vi "CR-导丝纤维毛发检测3参数读取.vi"(7 "error in (no error)":errorcluster caption="错误输入（无错误）", 10 "基路径":path) -> (0 "error out":errorcluster caption="错误输出", 1 "导丝纤维毛发检测3参数":T2={"Max Number"=11.0, "Curve Extraction Settings "={"Extraction Mode"=0, "Edge Threshold"=25, "Edge Filter Size"=1, "Min Length"=19, "Row Search Step Size"=5, "Col Search Step Size"=5, "Max Endpoint Gap"=10, "Closed"=FALSE, "Subpixel"=FALSE}, "Color Mode (Histogram 1)"=0, "Range (Threshold 1)"={"Lower value"=62.0, "Upper value"=255.0}, "Clamp Settings (Max Clamp 1)"={"Angle Range (+/-)"=10.0, "Edge Polarity"={"Start"=0, "End"=0}}, "Settings (Clamp (Rake) 1)"={"Contrast"=6, "Filter width"=5, "Steepness"=2, "Subsampling Ratio"=5, "Show Search Area"=TRUE, "Show Search Lines"=TRUE, "Show Edges Found"=TRUE, "Show Result"=TRUE}} {"Clamp Settings (Max Clamp 1)"."Edge Polarity"."Start" items=["Any", "Rising", "Falling"]; "Clamp Settings (Max Clamp 1)"."Edge Polarity"."End" items=["Any", "Rising", "Falling"]; "Color Mode (Histogram 1)" items=["RGB", "HSL", "HSV", "HSI"]; "Curve Extraction Settings"."Extraction Mode" items=["Normal", "Uniform Regions"]; "Curve Extraction Settings"."Edge Filter Size" items=["Fine", "Normal", "Contour Tracing"]; "Curve Extraction Settings"."Max Endpoint Gap" min=0; "Curve Extraction Settings"."Col Search Step Size" min=1 max=255 step=1; "Curve Extraction Settings"."Row Search Step Size" min=1 max=255 step=1; "Curve Extraction Settings"."Min Length" min=0; "Curve Extraction Settings"."Edge Threshold" min=1 max=350 step=1}, 2 "导丝纤维毛发检测3基础参数":T3={"IsNorImage"=TRUE, "Exposure Values"=100289, "ImagePath"=path "C:/Users/hedongpo/Desktop/514-hdp/Alignment Assemble System/Test Picture/B/3.bmp"} caption="参数界面" {"Exposure Values" scale=0.0..200000.0})   [LabVIEW 2017]
uses:
  <vilib>/vision/Pattern Matching.llb/IMAQ Curve Parameters.ctl
  <vilib>/Utility/xml.llb/Read From XML File(string).vi
  Global System.vi
panel:
  # "UI电源线反面标签1基础参数"
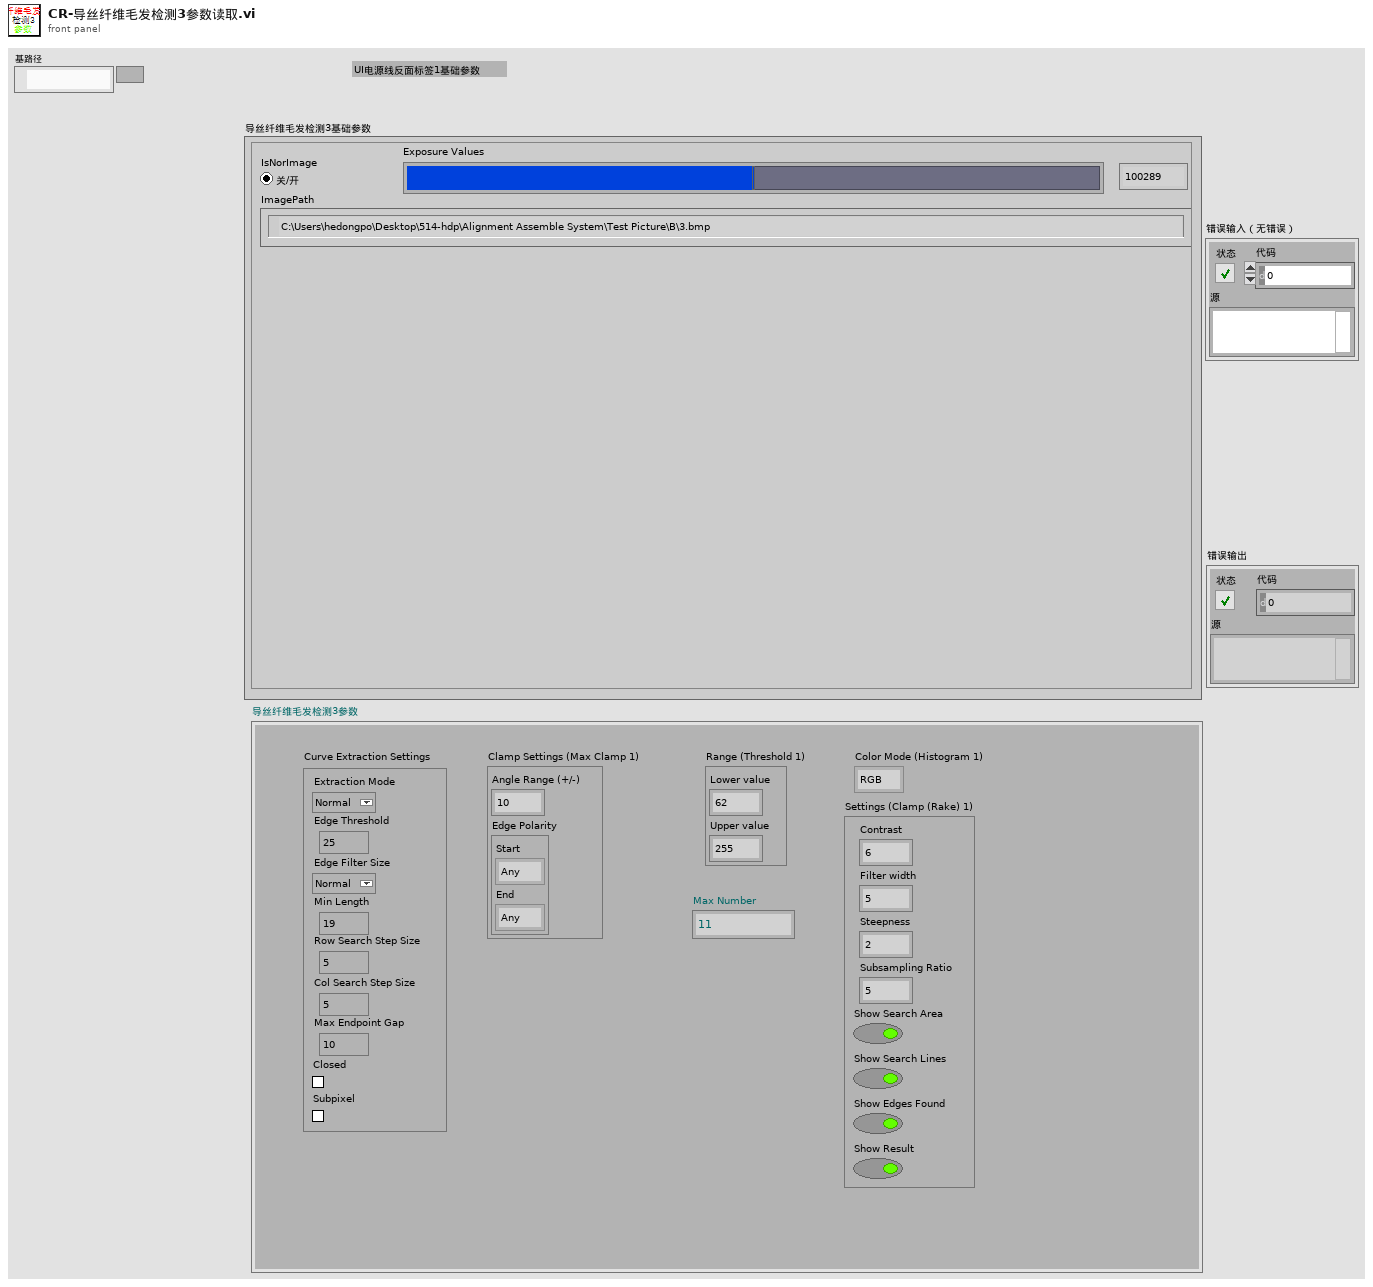
[diagram p1: front panel]
types:
  T1 = typedef "IMAQ Curve Parameters.ctl" = cluster{"Extraction Mode":u32, "Edge Threshold":i32, "Edge Filter Size":u32, "Min Length":i32, "Row Search Step Size":i32, "Col Search Step Size":i32, "Max Endpoint Gap":i32, "Closed":bool, "Subpixel":bool}
  T2 = cluster{"Max Number":sgl, "Curve Extraction Settings ":T1, "Color Mode (Histogram 1)":u16, "Range (Threshold 1)":cluster{"Lower value":sgl, "Upper value":sgl}, "Clamp Settings (Max Clamp 1)":cluster{"Angle Range (+/-)":dbl, "Edge Polarity":cluster{"Start":u32, "End":u32}}, "Settings (Clamp (Rake) 1)":cluster{"Contrast":i32, "Filter width":i32, "Steepness":i32, "Subsampling Ratio":u32, "Show Search Area":bool, "Show Search Lines":bool, "Show Edges Found":bool, "Show Result":bool}}
  T3 = cluster{"IsNorImage":bool, "Exposure Values":u32, "ImagePath":path}
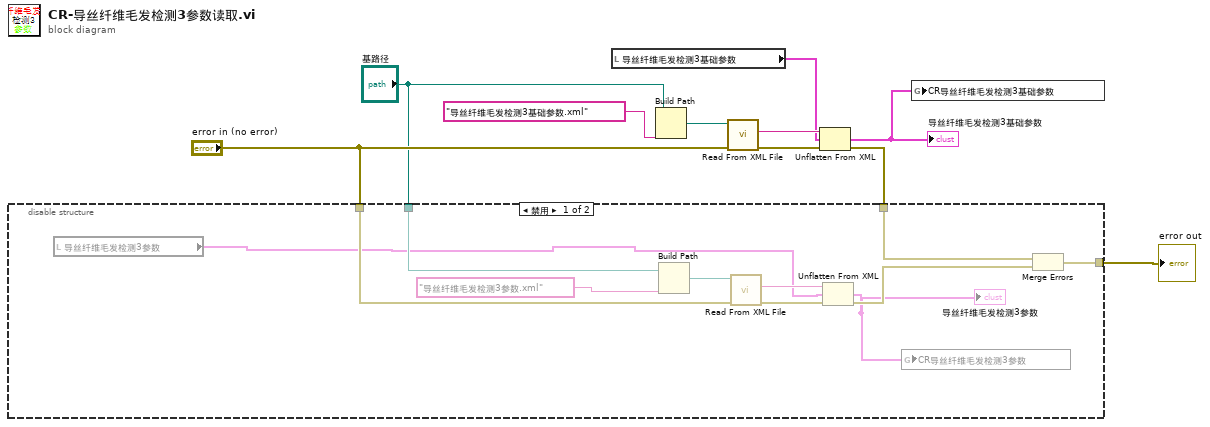
[diagram p0: block diagram]
diagram:
  n1 = local read "导丝纤维毛发检测3基础参数"() -> (w8:T3)
  n2 = Build Path(base path="基路径", name or relative path="导丝纤维毛发检测3基础参数.xml" ("名称或相对路径")) -> (appended path=w10:path)
  n3 = call-poly <vilib>:"Read From XML File.vi"("error in (no error)"="error in (no error)", "XML File Path"=w10) -> ("error out"=w6:errorcluster, "XML Elements"=w9:string)  [unwired: 7 in, 1 out]
  n4 = Unflatten From XML(xml string=w9, type=w8, error in (no error)=w6) -> (value=w1:T3, error out=w5:errorcluster)
  "导丝纤维毛发检测3基础参数" <- w1
  n5 = disable-structure shown="禁用" {
    disable-tunnel: "error in (no error)" -> [w19 _]
    disable-tunnel: w5 -> [w18 _]
    disable-tunnel: [w15 _] -> w4
    disable-tunnel: "基路径" -> [w14 _]
    frame Disabled {
      n6 = local read "导丝纤维毛发检测3参数"() -> (w13:T2)
      n7 = Build Path(base path=w14, name or relative path="导丝纤维毛发检测3参数.xml" ("名称或相对路径")) -> (appended path=w20:path)
      n8 = call-poly <vilib>:"Read From XML File.vi"("error in (no error)"=w19, "XML File Path"=w20) -> ("error out"=w17:errorcluster, "XML Elements"=w21:string)  [unwired: 7 in, 1 out]
      n9 = Unflatten From XML(xml string=w21, type=w13, error in (no error)=w17) -> (value=w11:T2, error out=w16:errorcluster)
      "导丝纤维毛发检测3参数" <- w11
      n10 = global write "Global System.vi" "CR导丝纤维毛发检测3参数"(w11) -> ()
      n11 = Merge Errors(w18, w16) -> (w15:errorcluster)
    }
    frame Enabled {
    }
  }
  "error out" <- w4
  n12 = global write "Global System.vi" "CR导丝纤维毛发检测3基础参数"(w1) -> ()
